vi "Get Camera Position.vi"(10 "Odometry Data":dbl[](array[numeric]), 11 "Camera Position":T1) -> (1 "Up Direction":cluster{"index":sgl, "index":sgl, "index":sgl}, 2 "Target":cluster{"DBL":dbl, "DBL":dbl, "index":sgl}, 3 "Camera Position":cluster{dbl, dbl, sgl})   [LabVIEW 2017]
uses:
  <vilib>/Utility/miscctls.llb/LV3DPointTypeDef.ctl
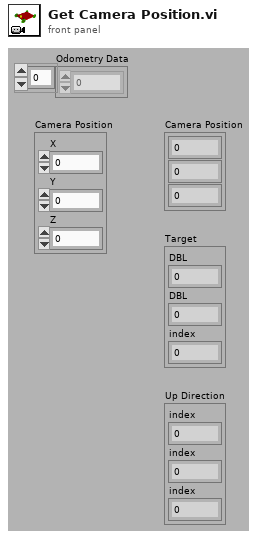
[diagram p1: front panel]
types:
  T1 = typedef "LV3DPointTypeDef.ctl" = cluster{"X":sgl, "Y":sgl, "Z":sgl}
  T2 = cluster{"Numeric":dbl, "Numeric":dbl, "index":sgl}
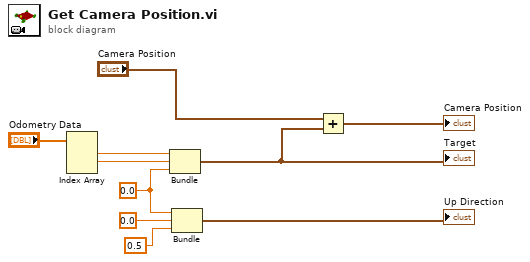
[diagram p0: block diagram]
diagram:
  w6 = sgl 0.0 ("index")
  n1 = Index Array(array="Odometry Data") -> (element #1=w2:dbl, element #2=w1:dbl)  [unwired: 3 in, 1 out]
  n2 = Bundle("Numeric"=w2, "Numeric"=w1, "index"=w6) -> (w9:T2)  [unwired: 1 in]
  "Target" <- w9
  n3 = Bundle("index"=w6, "index"=sgl 0.0, "index"=sgl 0.5) -> (→"Up Direction":cluster{"index":sgl, "index":sgl, "index":sgl})  [unwired: 1 in]
  n4 = Add(x="Camera Position", y=w9) -> (x+y=→"Camera Position":cluster{dbl, dbl, sgl})
